vi "QuickDrop Launch Window.vi"(10 "VI":string, 11 "App Refnum":refnum<vi>) -> ()   [LabVIEW 2018]
uses:
  <vilib>/Utility/QuickDropSupport/QuickDrop Plugin Data ver1.ctl
  <vilib>/Utility/miscctls.llb/LVRectTypeDef.ctl
  <vilib>/event_ctls.llb/eventvkey.ctl
  QuickDrop Shortcut Config.vi
  <resource>/dialog/lvconfig.llb/LV Config Write String.vi
  <resource>/dialog/lvconfig.llb/LV Config Read String.vi
  <helpdir>/_LaunchHelp.vi
  Find Project Items.vi
  <resource>/dialog/lvconfig.llb/LV Config Read Boolean.vi
  QuickDrop Get QDKS Mappings.vi
  <vilib>/UDC/API_Files/UDCCountUsage.vi
  <vilib>/UDC/niceiplib.lvlib
  <resource>/dialog/lvconfig.llb/LV Config Write Boolean.vi
  Load Default QD Object Shortcuts.vi
  <vilib>/UDC/API_Files/UDCLogFeatureUsage.vi
panel:
  in  "Object Name":string(combo)
  out "context help name":string
  in  "Waiting Msg":string[](array[string])=["Populating List... Please Wait"]
  out "Shortcuts":string[](array[string])
  in  "Done":bool
  in  "Name Match List":i32(listbox)
  in  "Help":bool
  in  "Configure":bool
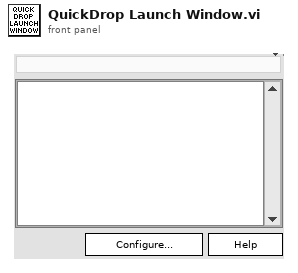
[diagram p1: front panel]
types:
  T1 = enum32{"Invalid", "Standard", "Closed", "Hidden", "Minimized", "Maximized"}
  T2 = cluster{"Left":i16, "Top":i16, "Right":i16, "Bottom":i16}
  T3 = typedef "LVAllMonitorsDisplayTypeDef.ctl" = cluster{"Bounds":cluster{"Left":i16, "Top":i16, "Right":i16, "Bottom":i16}, "Depth":i16}[]
  T4 = typedef "QuickDrop Plugin Data ver1.ctl" = cluster{"FP.IsFrontMost?":bool, "Project VI Path":path, "Palette Object Name":string}
  T5 = typedef "LVRectTypeDef.ctl" = cluster{"Left":i16, "Top":i16, "Right":i16, "Bottom":i16}
  T6 = typedef "eventvkey.ctl" = enum16{"ASCII", "Enter", "Return", "Shift", "Ctrl", "Alt", "Cmd", "Opt", "Caps", "NumLock", "Clear", "Break", "Up", "Down", "Left", "Right", "Insert", "Delete", "Home", "End", "PageUp", "PageDown", "Escape", "Help", "Pause", "ScrollLock", "F1", "F2", "F3", "F4", "F5", "F6", "F7", "F8", "F9", "F10", "F11", "F12", "F13", "F14", "F15", "F16", "F17", "F18", "F19", "F20", "F21", "F22", "F23", "F24", "Play", "VolumeUp", "VolumeDown", "Mute", "Two Byte Char"}
  T7 = cluster{"Shift":bool, "Ctrl":bool, "Alt":bool, "Cmd":bool, "Opt":bool}
  T8 = typedef "LVPoint32TypeDef.ctl" = cluster{"Horizontal":i32, "Vertical":i32}
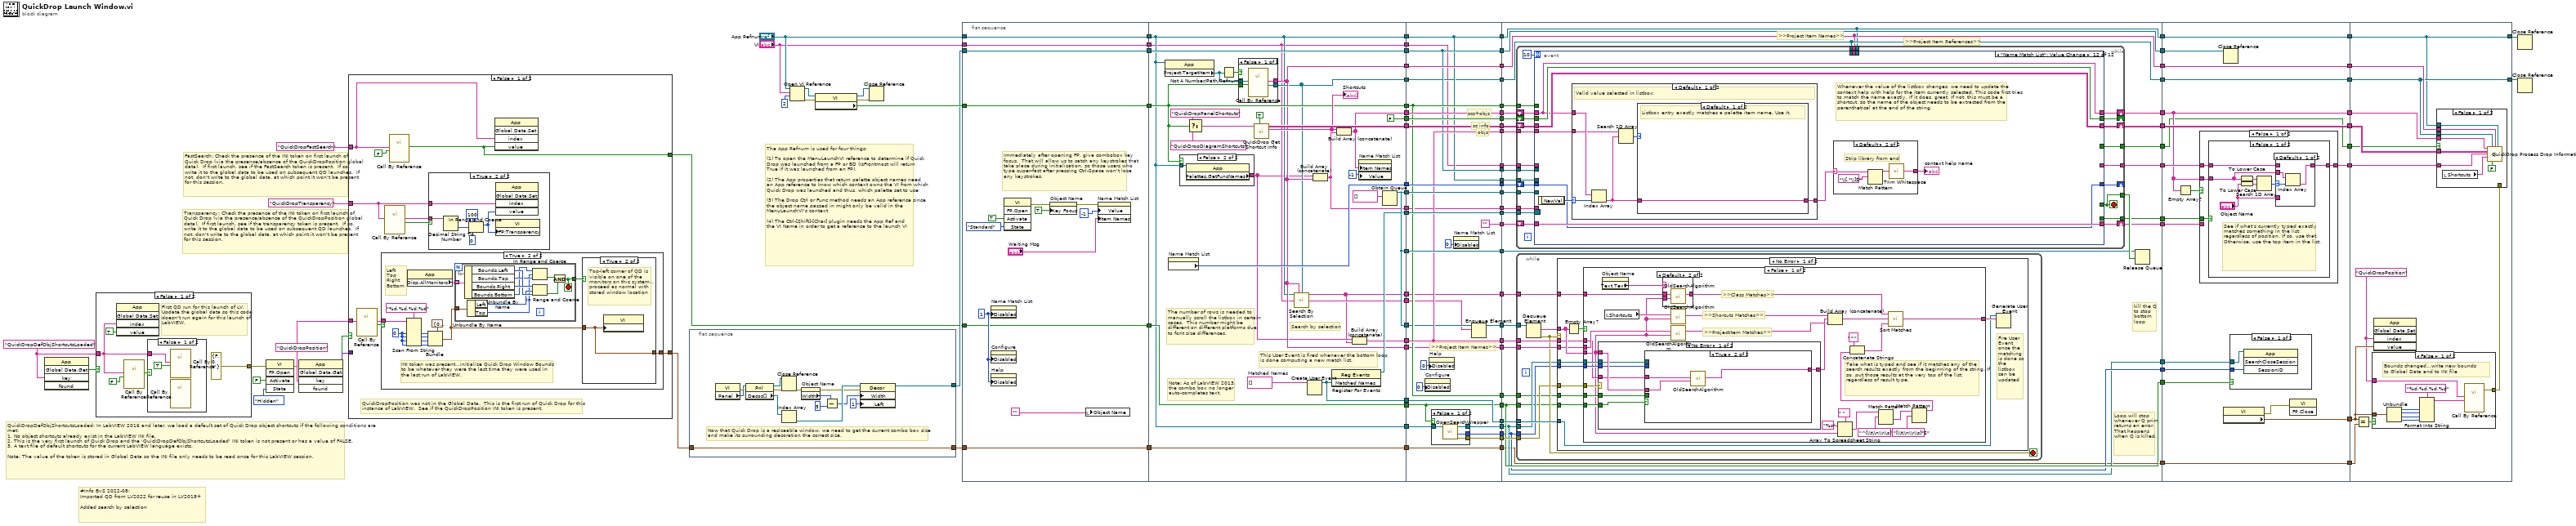
[diagram p0: block diagram]
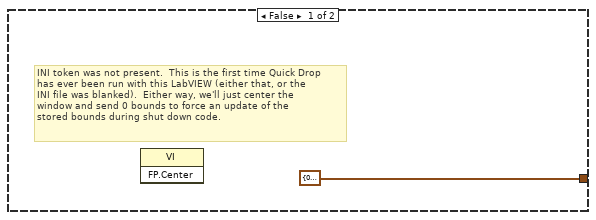
[diagram p5: hidden frame]
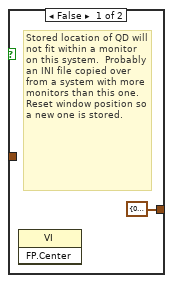
[diagram p6: hidden frame]
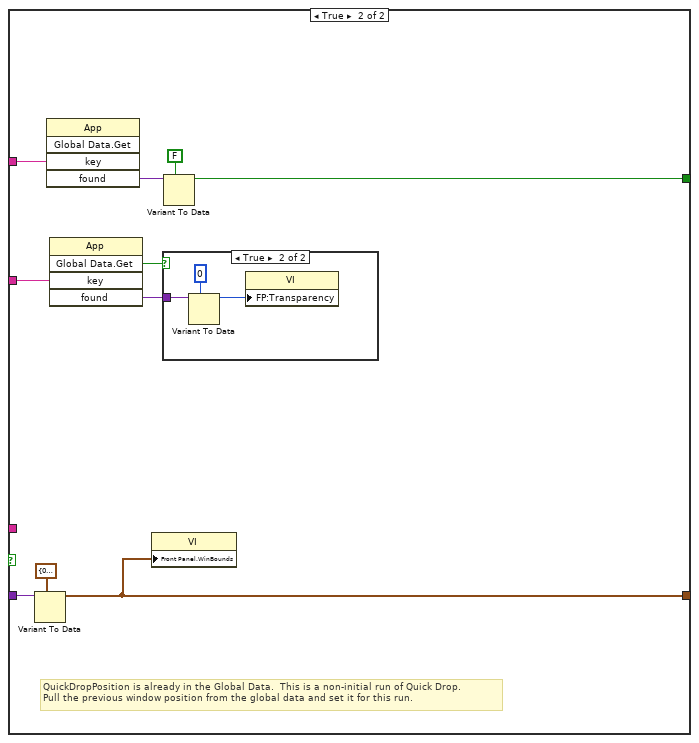
[diagram p7: hidden frame]
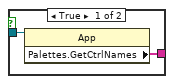
[diagram p10: hidden frame]
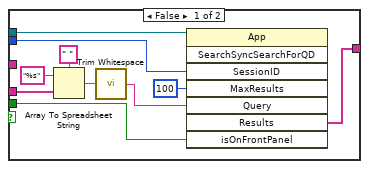
[diagram p13: hidden frame]
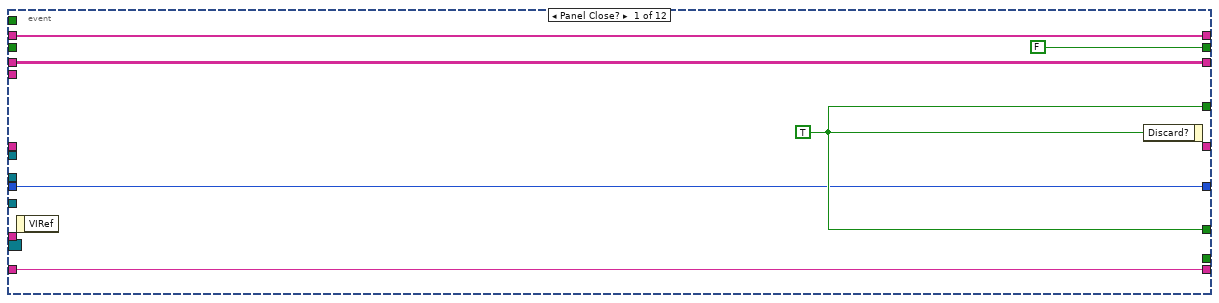
[diagram p17: hidden frame]
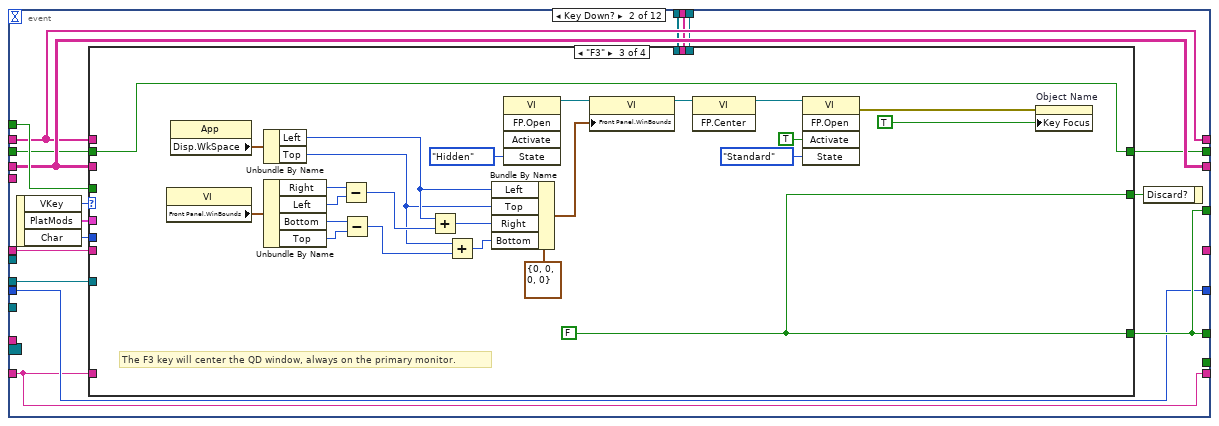
[diagram p18: hidden frame]
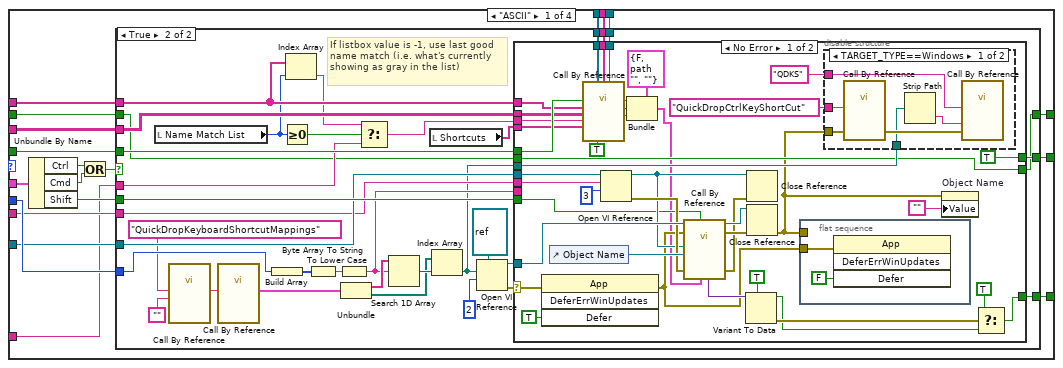
[diagram p19: hidden frame]
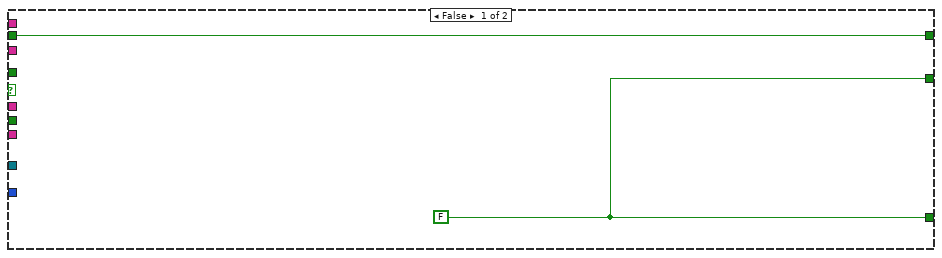
[diagram p20: hidden frame]
diagram:
  w6 = "QuickDropDefObjShortcutsLoaded" ("Name")
  w63 = "QuickDropPosition" ("Name")
  # "#Info BvS 2022-08:\nImported QD from LV2022 for reuse in LV2018+\n\nAdded search by selection"
  # "QuickDropDefObjShortcutsLoaded: In LabVIEW 2016 and later, we load a default set of Quick Drop object shortcuts if the following conditions are met:\n1. No object shortcuts already exist in the LabVIEW INI file.\n2. This is the very first launch of Quick Drop and the 'QuickDropDefObjShortcutsLoaded' INI token is not present or has a value of FALSE.\n3. A text file of default shortcuts for the current LabVIEW language exists.\n\nNote: The value of the token is stored in Global Data so the INI file only needs to be read once for this LabVIEW session."
  # "FastSearch: Check the presence of the INI token on first launch of Quick Drop (via the presence/absence of the QuickDropPosition global data).  If first launch, see if the FastSearch token is present.  If so, write it to the global data to be used on subsequent QD launches.  If not, don't write to the global data, at which point it won't be present for this session."
  # "Transparency: Check the presence of the INI token on first launch of Quick Drop (via the presence/absence of the QuickDropPosition global data).  If first launch, see if the transparency token is present.  If so, write it to the global data to be used on subsequent QD launches.  If not, don't write to the global data, at which point it won't be present for this session."
  # "The App Refnum is used for four things:\n\n(1) To open the MenuLaunchVI reference to determine if Quick Drop was launched from a FP or BD (IsFrontmost will return True if it was launched from an FP).\n\n(2) The App properties that return palette object names need an App reference to know which context owns the VI from which Quick Drop was launched and thus, which palette set to use\n\n(3) The Drop Ctrl or Func method needs an App reference since the object name passed in might only be valid in the MenuLaunchVI's context \n\n(4) The Ctrl-[Shift]-[Char] plugin needs the App Ref and\nthe VI Name in order to get a reference to the launch VI"
  n1 = invoke class="App" method="Global Data.Get"("key"=w6) -> ("GlobalData:Get"=w5:bool)  [unwired: 4 in, 4 out]
  n2 = case shown="False" w5 {
    tunnel: w6 -> [w107 _]
    tunnel: [errorcluster {"status"=FALSE, "code"=0, "source"=""} ("error constant") _] -> w4
    frame False {
      # "First QD run for this launch of LV. Update the global data so this code doesn't run again for this launch of LabVIEW."
      n3 = invoke class="App" method="Global Data.Set"("index"=w107, "value"=TRUE) -> ()  [unwired: 3 in, 5 out]
      n4 = call-by-ref "?"("default value"=FALSE, "key"=w107) -> ("value"=w109:bool)  [unwired: 5 in, 4 out]
      n5 = case shown="False" w109 {
        tunnel: w107 -> [w113 _]
        frame False {
          n6 = call-by-ref "?"("value"=TRUE, "key"=w113) -> ()  [unwired: 7 in, 3 out]
          n7 = call-by-ref "?"() -> ()  [unwired: 14 in, 2 out]
        }
        frame True {
          # "QD default object shortcut code has already been called once in the history of this LabVIEW. Do nothing."
        }
      }
    }
    frame True {
      # "This is the non-initial use of Quick Drop for this launch of LabVIEW. All the Quick Drop default object shortcut initialization stuff has already happened."
    }
  }
  n8 = invoke class="VI" method="FP.Open"(error in=w4, "Activate"=FALSE ("Activate?"), "State"=T1."Hidden") -> (error out=w26:errorcluster)  [unwired: 2 in, 4 out]
  n9 = invoke class="App" method="Global Data.Get"(error in=w26, "key"=w63) -> ("GlobalData:Get"=w10:bool, "found"=w64:variant)  [unwired: 3 in, 3 out]
  n10 = case shown="False" w10 {
    tunnel: w64 -> [_ w165]
    tunnel: [w123 w163] -> w25
    tunnel: w63 -> [w122 _]
    tunnel: "QuickDropTransparency" ("Name") -> [w117 w162]
    tunnel: "QuickDropFastSearch" ("Name") -> [w116 w159]
    tunnel: [w115 w156] -> w17
    frame False {
      # "QuickDropPosition was not in the Global Data.  This is the first run of Quick Drop for this\ninstance of LabVIEW.  See if the QuickDropPosition INI token is present."
      n11 = call-by-ref "?"("key"=w122) -> ("found?"=w121:bool, "value"=w120:string)  [unwired: 6 in, 3 out]
      n12 = case shown="True" w121 {
        tunnel: [T2 {"Left"=0, "Top"=0, "Right"=0, "Bottom"=0} ("Front Panel.PanelBounds") w131] -> w123
        tunnel: w120 -> [_ w142]
        frame False {
          # "INI token was not present.  This is the first time Quick Drop\nhas ever been run with this LabVIEW (either that, or the\nINI file was blanked).  Either way, we'll just center the\nwindow and send 0 bounds to force an update of the\nstored bounds during shut down code."
          n13 = invoke class="VI" method="FP.Center"() -> ()  [unwired: 3 in, 3 out]
        }
        frame True {
          w140 = i16 0 ("default value 1")
          # "Left\nTop\nRight\nBottom"
          # "INI token was present...initialize Quick Drop Window Bounds\nto be whatever they were the last time they were used in\nthe last run of LabVIEW."
          n14 = Scan From String(format string="%d,%d,%d,%d", input string=w142, default 1=w140, default 2=w140, default 3=w140, default 4=w140) -> (output 1=w139:i16, output 2=w138:i16, output 3=w137:i16, output 4=w136:i16)  [unwired: 2 in, 3 out]
          n15 = property class="App"() -> ("Disp.AllMonitors"=w134:T3)  [unwired: 2 in, 2 out]
          n16 = Bundle(cluster=T2 {"Left"=0, "Top"=0, "Right"=0, "Bottom"=0} ("Front Panel.PanelBounds"), "Left"=w139, "Top"=w138, "Right"=w137, "Bottom"=w136) -> (w133:T2)
          n17 = for {
            tunnel: w134 -> [w155] mode=indexing
            tunnel: w133 -> [w154]
            tunnel: [w145] -> w132
            stop <- w145 stop-if-true
            n18 = Unbundle By Name(w155) -> ("Bounds.Left"=w152:i16, "Bounds.Top"=w150:i16, "Bounds.Right"=w153:i16, "Bounds.Bottom"=w149:i16)
            n19 = Unbundle By Name(w154) -> ("Left"=w151:i16, "Top"=w148:i16)
            n20 = In Range and Coerce(upper limit=w149, x=w148, lower limit=w150) -> (In Range?=w147:bool)  [unwired: 1 out]
            n21 = In Range and Coerce(upper limit=w153, x=w151, lower limit=w152) -> (In Range?=w146:bool)  [unwired: 1 out]
            n22 = And(x=w147, y=w146) -> (x .and. y?=w145:bool)
          }
          n23 = case shown="True" w132 {
            tunnel: w133 -> [_ w144]
            tunnel: [T2 {"Left"=0, "Top"=0, "Right"=0, "Bottom"=0} ("Front Panel.PanelBounds") w144] -> w131
            frame False {
              # "Stored location of QD will not fit within a monitor on this system.  Probably an INI file copied over from a system with more monitors than this one.  Reset window position so a new one is stored."
              n24 = invoke class="VI" method="FP.Center"() -> ()  [unwired: 3 in, 3 out]
            }
            frame True {
              # "Top-left corner of QD is visible on one of the monitors on this system... proceed as normal with stored window location"
              n25 = property class="VI"("Front Panel.WinBounds"=w144) -> ()  [unwired: 2 in, 2 out]
            }
          }
        }
      }
      n26 = call-by-ref "?"("key"=w117) -> ("found?"=w119:bool, "value"=w118:string)  [unwired: 6 in, 3 out]
      n27 = call-by-ref "?"("default value"=FALSE, "key"=w116) -> ("value"=w115:bool)  [unwired: 5 in, 4 out]
      n28 = case shown="True" w119 {
        tunnel: w118 -> [_ w129]
        tunnel: w117 -> [_ w125]
        frame False {
        }
        frame True {
          n29 = Decimal String To Number(string=w129) -> (number=w128:i32)  [unwired: 2 in, 1 out]
          n30 = In Range and Coerce(upper limit=100 ("lower limit"), x=w128, lower limit=0) -> (coerced(x)=w124:i32)  [unwired: 1 out]
          n31 = invoke class="App" method="Global Data.Set"("index"=w125, "value"=w124) -> ()  [unwired: 3 in, 5 out]
          n32 = property class="VI"("FP:Transparency"=w124) -> ()  [unwired: 2 in, 2 out]
        }
      }
      n33 = invoke class="App" method="Global Data.Set"("index"=w116, "value"=w115) -> ()  [unwired: 3 in, 5 out]
    }
    frame True {
      # "QuickDropPosition is already in the Global Data.  This is a non-initial run of Quick Drop.\nPull the previous window position from the global data and set it for this run."
      n34 = Variant To Data(type=T2 {"Left"=0, "Top"=0, "Right"=0, "Bottom"=0} ("Front Panel.PanelBounds"), Variant=w165) -> (data=w163:T2)  [unwired: 1 in, 1 out]
      n35 = invoke class="App" method="Global Data.Get"("key"=w159) -> ("found"=w158:variant)  [unwired: 4 in, 4 out]
      n36 = invoke class="App" method="Global Data.Get"("key"=w162) -> ("GlobalData:Get"=w161:bool, "found"=w160:variant)  [unwired: 4 in, 3 out]
      n37 = property class="VI"("Front Panel.WinBounds"=w163) -> ()  [unwired: 2 in, 2 out]
      n38 = case shown="True" w161 {
        tunnel: w160 -> [_ w168]
        frame False {
        }
        frame True {
          n39 = Variant To Data(type=0 ("lower limit"), Variant=w168) -> (data=w166:i32)  [unwired: 1 in, 1 out]
          n40 = property class="VI"("FP:Transparency"=w166) -> ()  [unwired: 2 in, 2 out]
        }
      }
      n41 = Variant To Data(type=FALSE, Variant=w158) -> (data=w156:bool)  [unwired: 1 in, 1 out]
    }
  }
  n42 = flat-sequence {
    tunnel: [w182] -> w24
    tunnel: w25 -> [w182]
    tunnel: [w170] -> w23
    frame #0 {
      # "Now that Quick Drop is a resizeable window, we need to get the current combo box size\nand make its surrounding decoration the correct size."
      n43 = property class="VI"() -> (error out=w171:errorcluster, "Panel"=w172:refnum<vi>)  [unwired: 2 in, 1 out]
      n44 = property class="Pnl"(reference=w172, error in=w171) -> (reference out=w174:refnum<vi>, error out=w173:errorcluster, "Decos[]"=w179:refnum<vi>[])
      n45 = Index Array(array=w179) -> (element=w181:refnum<vi>)  [unwired: 1 in]
      n46 = Close Reference(reference=w174, error in (no error)=w173) -> (error out=w175:errorcluster)
      n47 = property on="Object Name" class="CmbBox"(error in=w175) -> (error out=w180:errorcluster, "Width"=w176:u32)  [unwired: 1 in, 1 out]
      n48 = Subtract(x=w176, y=u32 5) -> (x-y=w178:u32)
      n49 = property class="Decor"(reference=w181, error in=w180, "Width"=w178, "Left"=1 ("Position:Left")) -> (reference out=w170:refnum<vi>)  [unwired: 1 out]
    }
  }
  n50 = Open VI Reference(application reference (local)="App Refnum", vi path="VI", options=2) -> (vi reference=w75:refnum<vi>, error out=w65:errorcluster)  [unwired: 1 in, 2 out]
  n51 = property class="VI"(reference=w75, error in=w65) -> (reference out=w73:refnum<vi>, error out=w74:errorcluster, "Front Panel.IsFrontmost"=w72:bool)
  n52 = Close Reference(reference=w73, error in (no error)=w74) -> ()  [unwired: 1 out]
  n53 = flat-sequence {
    tunnel: w24 -> [w195]
    tunnel: w72 -> [w196]
    tunnel: "App Refnum" -> [w197]
    tunnel: [w197] -> w54
    tunnel: [w196] -> w53
    tunnel: [w195] -> w52
    tunnel: [w189] -> w35
    tunnel: "VI" -> [w189]
    tunnel: [w185] -> w29
    tunnel: w23 -> [w185]
    tunnel: [w184] -> w18
    tunnel: w17 -> [w184]
    tunnel: [w216] -> w106
    tunnel: [FALSE] -> w104
    tunnel: [w226] -> w102
    tunnel: [w226] -> w100
    tunnel: [w205] -> w98
    tunnel: [w226] -> w96
    tunnel: [w201] -> w94
    tunnel: [w224] -> w92
    tunnel: [w223] -> w90
    tunnel: [w222] -> w88
    tunnel: [w210] -> w84
    tunnel: [w217] -> w82
    tunnel: [w203] -> w70
    tunnel: [w213] -> w62
    tunnel: w54 -> [w203]
    tunnel: w53 -> [w210]
    tunnel: w52 -> [w213]
    tunnel: [w204] -> w50
    tunnel: [w205] -> w46
    tunnel: [w203] -> w42
    tunnel: w35 -> [w202]
    tunnel: [w202] -> w32
    tunnel: [w209] -> w30
    tunnel: w29 -> [w208]
    tunnel: [w208] -> w28
    tunnel: w18 -> [w207]
    tunnel: [w207] -> w15
    tunnel: [w198] -> w2
    tunnel: [w199] -> w1
    tunnel: w106 -> [w266]
    tunnel: [w266] -> w105
    tunnel: w104 -> [w265]
    tunnel: [w265] -> w103
    tunnel: w102 -> [w264]
    tunnel: [w264] -> w101
    tunnel: w100 -> [w243]
    tunnel: [w242] -> w99
    tunnel: w98 -> [w240]
    tunnel: [w240] -> w97
    tunnel: w96 -> [w263]
    tunnel: [w263] -> w95
    tunnel: w94 -> [w259]
    tunnel: [w259] -> w93
    tunnel: w92 -> [w262]
    tunnel: [w262] -> w91
    tunnel: w90 -> [w246]
    tunnel: [w246] -> w89
    tunnel: w88 -> [w261]
    tunnel: [w261] -> w87
    tunnel: [w259] -> w86
    tunnel: [w249] -> w85
    tunnel: w84 -> [w249]
    tunnel: [w260] -> w83
    tunnel: w82 -> [w260]
    tunnel: [w241] -> w71
    tunnel: w70 -> [w241]
    tunnel: [w241] -> w67
    tunnel: w62 -> [w258]
    tunnel: [w258] -> w59
    tunnel: w50 -> [w239]
    tunnel: [w239] -> w49
    tunnel: w46 -> [w254]
    tunnel: [w254] -> w45
    tunnel: w42 -> [w253]
    tunnel: [w252] -> w41
    tunnel: [w251] -> w40
    tunnel: [w250] -> w39
    tunnel: [w249] -> w38
    tunnel: [w238] -> w33
    tunnel: w32 -> [w238]
    tunnel: [w248] -> w31
    tunnel: w30 -> [w248]
    tunnel: w28 -> [w247]
    tunnel: [w247] -> w27
    tunnel: [w247] -> w21
    tunnel: [w245] -> w16
    tunnel: w15 -> [w245]
    tunnel: [""] -> w9
    tunnel: [w237] -> w3
    tunnel: w2 -> [w237]
    tunnel: w1 -> [w236]
    tunnel: w105 -> [w306]
    tunnel: w103 -> [w305]
    tunnel: w101 -> [w304]
    tunnel: w99 -> [w303]
    tunnel: w97 -> [w302]
    tunnel: w95 -> [w300]
    tunnel: w93 -> [w299]
    tunnel: w91 -> [w298]
    tunnel: w89 -> [w297]
    tunnel: w87 -> [w296]
    tunnel: [w295] -> w81
    tunnel: [w294] -> w79
    tunnel: w86 -> [w293]
    tunnel: w85 -> [w292]
    tunnel: w83 -> [w291]
    tunnel: [w290] -> w77
    tunnel: w71 -> [w275]
    tunnel: [w275] -> w68
    tunnel: w67 -> [w289]
    tunnel: [w279] -> w60
    tunnel: w59 -> [w279]
    tunnel: [w288] -> w55
    tunnel: w49 -> [w277]
    tunnel: [w277] -> w48
    tunnel: w45 -> [w276]
    tunnel: [w276] -> w44
    tunnel: w41 -> [w280]
    tunnel: w40 -> [w281]
    tunnel: w39 -> [w287]
    tunnel: w38 -> [w286]
    tunnel: [w280] -> w37
    tunnel: [w281] -> w36
    tunnel: w33 -> [w285]
    tunnel: w31 -> [w284]
    tunnel: w27 -> [w283]
    tunnel: [w278] -> w22
    tunnel: w21 -> [w278]
    tunnel: w16 -> [w282]
    tunnel: [w282] -> w14
    tunnel: w9 -> [w274]
    tunnel: [w273] -> w8
    tunnel: [w272] -> w7
    tunnel: w3 -> [w271]
    tunnel: w81 -> [w908]
    tunnel: [w908] -> w80
    tunnel: w79 -> [w911]
    tunnel: [w910] -> w78
    tunnel: w77 -> [w922]
    tunnel: [w922] -> w76
    tunnel: [w921] -> w69
    tunnel: w68 -> [w921]
    tunnel: [w920] -> w61
    tunnel: w60 -> [w920]
    tunnel: [w919] -> w58
    tunnel: w55 -> [w909]
    tunnel: w48 -> [w917]
    tunnel: [w917] -> w47
    tunnel: w44 -> [w916]
    tunnel: [w916] -> w43
    tunnel: w37 -> [w915]
    tunnel: w36 -> [w914]
    tunnel: w22 -> [w913]
    tunnel: w14 -> [w912]
    tunnel: [w909] -> w13
    tunnel: w8 -> [w906]
    tunnel: w7 -> [w905]
    tunnel: w80 -> [w948]
    tunnel: w78 -> [w953]
    tunnel: w76 -> [w952]
    tunnel: w69 -> [w944]
    tunnel: w61 -> [w951]
    tunnel: w58 -> [w943]
    tunnel: w47 -> [w945]
    tunnel: w43 -> [w949]
    tunnel: w13 -> [w946]
    tunnel: [w945] -> w12
    tunnel: [w944] -> w11
    frame #0 {
      w191 = u8 1 ("Disabled")
      # "Immediately after opening FP, give combobox key focus.  That will allow us to catch any keystrokes that take place during initialization, so those users who type super-fast after pressing Ctrl-Space won't lose any keystrokes."
      n54 = property on="Name Match List" class="LstBox (strict)"("Disabled"=w191) -> ()  [unwired: 2 in, 2 out]
      n55 = property on="Configure" class="Bool"("Disabled"=w191) -> ()  [unwired: 2 in, 2 out]
      n56 = property on="Help" class="Bool"("Disabled"=w191) -> ()  [unwired: 2 in, 2 out]
      n57 = invoke class="VI" method="FP.Open"("Activate"=TRUE ("Activate?"), "State"=T1."Standard") -> (error out=w187:errorcluster)  [unwired: 3 in, 4 out]
      n58 = property on="Object Name" class="CmbBox"(error in=w187, "Key Focus"=TRUE) -> (error out=w186:errorcluster)  [unwired: 1 in, 1 out]
      n59 = local write "Object Name"("") -> ()
      n60 = property on="Name Match List" class="LstBox (strict)"(error in=w186, "Value"=-1 ("Name Match List"), "Item Names"="Waiting Msg") -> ()  [unwired: 1 in, 2 out]
    }
    frame #1 {
      w225 = string[] []  # Matched Names
      # "Search by selection"
      # "Note: As of LabVIEW 2013,\nthe combo box no longer\nauto-completes text."
      # "The number of rows is needed to manually scroll the listbox in certain cases.  This number might be different on different platforms due to font size differences."
      # "This User Event is fired whenever the bottom loop is done computing a new match list."
      n61 = property class="App"(reference=w203) -> ("Project.TargetItem"=w206:refnum<vi>)  [unwired: 1 in, 2 out]
      n62 = property on="Name Match List" class="LstBox (strict)"() -> ("Number of Rows"=w222:u32)  [unwired: 2 in, 2 out]
      n63 = case shown="False" w210 {
        tunnel: [w233 w235] -> w200
        tunnel: w203 -> [w232 w234]
        frame True {
          n64 = property class="App"(reference=w232) -> ("Palettes.GetCtrlNames"=w233:string[])  [unwired: 1 in, 2 out]
        }
        frame False {
          n65 = property class="App"(reference=w234) -> ("Palettes.GetFuncNames"=w235:string[])  [unwired: 1 in, 2 out]
        }
      }
      n66 = Select(t="QuickDropPanelShortcuts" ("Name"), s=w210, f="QuickDropDiagramShortcuts" ("Name")) -> (s? t:f=w219:string)
      n67 = Not A Number/Path/Refnum?(number/path/refnum=w206) -> (NaN/Path/Refnum?=w211:bool)
      n68 = case shown="False" w211 {
        tunnel: w206 -> [w228 _]
        tunnel: w210 -> [w231 _]
        tunnel: [w230 _] -> w205
        tunnel: [w229 _] -> w204
        frame False {
          n69 = call-by-ref "?"("Panel?"=w231, "Target Item"=w228) -> ("Project Item Ref"=w229:refnum<vi>[], "Hierarchy"=w230:string[])  [unwired: 10 in, 2 out]
        }
        frame True {
        }
      }
      n70 = call "QuickDrop Get Shortcut Info.vi"("Generate Listbox Strings?"=TRUE, "Shortcut Type"=w219) -> ("Listbox Strings"=w215:string[], "Shortcut Info"=w217:string[][])  [unwired: 1 in, 7 out]
      "Shortcuts" <- w215
      n71 = call "Search By Selection.vi"("App Refnum"=w203, "Project Item Names"=w205, "Project Item Refs"=w204, "VI"=w202) -> ("Class Item Names"=w198:string[], "Query terms"=w199:string[])  [unwired: 9 in, 1 out]
      n72 = Create User Event(user event datatype=w225) -> (user event=w223:refnum<user-event>)  [unwired: 1 in, 1 out]
      n73 = Build Array (concatenate)(w200, w205) -> (w209:string[])
      n74 = register-events(w223) -> (reference out=w224:refnum<event-registration>)  [unwired: 2 in, 1 out]
      n75 = Build Array (concatenate)(w215, w209) -> (w216:string[])
      n76 = Build Array (concatenate)(w200, w198) -> (w201:string[])
      n77 = property on="Name Match List" class="LstBox (strict)"("Item Names"=w216, "Value"=-1 ("Listbox")) -> ()  [unwired: 2 in, 2 out]
      n78 = Obtain Queue(element data type=string[] []) -> (queue out=w226:refnum<queue>)  [unwired: 3 in, 3 out]
    }
    frame #2 {
      # ">>Project Item Names>>"
      # "objs"
      # "sc info"
      # "scs+objs"
      n79 = property on="Configure" class="Bool"("Disabled"=u8 0) -> ()  [unwired: 2 in, 2 out]
      n80 = property on="Help" class="Bool"("Disabled"=u8 0) -> ()  [unwired: 2 in, 2 out]
      n81 = case shown="False" w245 {
        tunnel: w253 -> [w270 _]
        tunnel: [w269 _] -> w252
        tunnel: [w268 _] -> w251
        tunnel: [w267 _] -> w250
        frame False {
          n82 = call "OpenSearchWrapper.vi"("App Refnum"=w270) -> ("error out"=w267:errorcluster, "Session ID out"=w268:u32, "App Refnum Out"=w269:refnum<vi>)  [unwired: 8 in]
        }
        frame True {
        }
      }
      n83 = property on="Name Match List" class="LstBox (strict)"("Disabled"=u8 0) -> ()  [unwired: 2 in, 2 out]
      n84 = Enqueue Element(queue=w243, element=w236) -> (queue out=w242:refnum<queue>)  [unwired: 2 in, 2 out]
    }
    frame #3 {
      # ">>Project Item Names>>"
      # ">>Project Item References>>"
      # "Loop will stop whenever Q prim returns an error.  That happens when Q is killed."
      # "kill the Q\nto stop\nbottom\nloop"
      n85 = while {
        shift-right: [w406] -> w288
        shift-left: w306 -> [w407]
        shift-right: [w403] -> _
        shift-left: w305 -> [w404]
        tunnel: w304 -> [w402]
        tunnel: [w401] -> w301
        tunnel: w298 -> [w400]
        tunnel: [w398] -> w295
        tunnel: [w397] -> w294
        tunnel: w293 -> [w396]
        tunnel: w292 -> [w395]
        shift-right: [w393] -> w290
        shift-left: w291 -> [w394]
        tunnel: w289 -> [w392]
        tunnel: w285 -> [w391]
        tunnel: w284 -> [w390]
        tunnel: w283 -> [w389]
        shift-right: [w388] -> _
        shift-left: w296 -> [w399]
        tunnel: w277 -> [w387]
        tunnel: w276 -> [w386]
        tunnel: w275 -> [w385]
        shift-right: [w383] -> w273
        shift-left: w274 -> [w384]
        tunnel: [w382] -> w272
        stop <- w401 stop-if-true
        n86 = event shown="[11] \"Name Match List\": Value Change" {
          selector: w400 -> [_ _ _ _ _ _ _ _ _ _ _ _]
          dyn-events: _ -> [_ _ _ _ _ _ _ _ _ _ _ _]
          timeout: 10 -> [_ _ _ _ _ _ _ _ _ _ _ _]
          tunnel: [w411 w430 TRUE ("Discard?") w591 w609 _ _ _ _ _ _ _] -> w401
          tunnel: w407 -> [w413 w420 w579 w590 w602 w620 w626 w660 w793 _ w876 w880]
          tunnel: [w413 w420 w579 w590 w602 w620 w625 w660 w793 w820 w876 w880] -> w406
          tunnel: w404 -> [_ w415 _ _ _ w619 _ _ w790 w815 w875 w883]
          tunnel: [FALSE w414 FALSE FALSE FALSE w619 FALSE w648 FALSE w815 w875 w883] -> w403
          tunnel: w402 -> [_ _ _ _ _ _ _ _ w791 _ _ _]
          tunnel: w399 -> [w409 w424 w580 w586 w605 w615 w623 w659 w788 w828 _ w879]
          tunnel: [w411 w430 FALSE ("Discard?") FALSE ("Discard?") FALSE ("Discard?") _ _ _ _ _ _ _] -> w398
          tunnel: [_ _ w578 w595 w603 _ _ _ _ _ _ _] -> w397
          tunnel: w396 -> [_ _ _ _ _ _ w632 _ _ _ _ w881]
          tunnel: w395 -> [_ w423 _ _ _ _ w633 _ _ _ _ _]
          tunnel: w394 -> [w410 w421 w581 w596 w606 w618 w627 w662 w789 w821 w874 w882]
          tunnel: [w410 w421 w581 w596 w606 w618 w629 w662 w789 w821 w874 w882] -> w393
          tunnel: w392 -> [_ w426 _ _ _ _ w630 _ _ _ _ _]
          tunnel: w391 -> [_ w425 _ _ _ _ _ _ _ _ _ _]
          tunnel: w390 -> [_ _ _ _ _ _ w624 _ _ _ _ _]
          tunnel: w389 -> [_ _ _ _ _ _ _ _ _ _ w870 _]
          tunnel: [w409 w424 w580 w586 w605 w615 w623 w659 w788 w828 w867 w879] -> w388
          tunnel: w387 -> [_ w419 _ _ _ _ _ _ _ _ _ _]
          tunnel: w386 -> [_ w418 _ _ _ _ _ _ _ _ _ _]
          tunnel: w385 -> [_ w417 _ _ _ _ _ _ _ _ _ _]
          tunnel: w384 -> [w408 w416 w577 w585 w601 w614 w622 w649 w787 w826 w865 w885]
          tunnel: [w408 w416 w577 w585 w601 w614 w622 w649 w787 w816 w865 w885] -> w383
          tunnel: [_ _ w575 w584 w599 _ _ _ _ _ _ _] -> w382
          event Panel Close? {
            w411 = TRUE ("Discard?")
            n87 = event-data() -> ()  [unwired: 2 out]
            n88 = event-data("Discard?"=w411) -> ()  [unwired: 1 in, 1 out]
          }
          event Key Down? {
            n89 = event-data() -> ("VKey"=w429:T6, "PlatMods"=w428:T7, "Char"=w427:i16)  [unwired: 1 out]
            n90 = case shown="\"F3\"" w429 {
              tunnel: [w444 TRUE w571 w573] -> w430
              tunnel: w428 -> [w449 _ _ _]
              tunnel: w427 -> [w443 _ _ _]
              tunnel: w426 -> [w442 _ _ _]
              tunnel: w425 -> [w441 _ _ _]
              tunnel: w423 -> [w440 _ _ _]
              tunnel: [w439 FALSE w571 w573] -> w422
              tunnel: w421 -> [w438 _ _ _]
              tunnel: w420 -> [w437 _ _ _]
              tunnel: w419 -> [w436 _ _ _]
              tunnel: w418 -> [w435 _ _ _]
              tunnel: w417 -> [w434 _ _ _]
              tunnel: w416 -> [w433 _ _ _]
              tunnel: w415 -> [w432 w545 w548 w572]
              tunnel: [w431 w545 w548 w572] -> w414
              frame "ASCII" {
                n91 = Unbundle By Name(w449) -> ("Ctrl"=w448:bool, "Cmd"=w447:bool, "Shift"=w445:bool)
                n92 = Or(x=w448, y=w447) -> (x .or. y?=w446:bool)
                n93 = case shown="True" w446 {
                  tunnel: w445 -> [_ w480]
                  tunnel: [w451 w481] -> w444
                  tunnel: w443 -> [_ w465]
                  tunnel: w442 -> [_ w479]
                  tunnel: w441 -> [_ w478]
                  tunnel: w440 -> [_ w477]
                  tunnel: [w451 w476] -> w439
                  tunnel: w438 -> [_ w471]
                  tunnel: w437 -> [_ w466]
                  tunnel: w436 -> [_ w469]
                  tunnel: w435 -> [_ w468]
                  tunnel: w434 -> [_ w467]
                  tunnel: w433 -> [_ w456]
                  tunnel: w432 -> [w450 w453]
                  tunnel: [w450 w452] -> w431
                  frame False {
                    w451 = FALSE
                  }
                  frame True {
                    # "If listbox value is -1, use last good name match (i.e. what's currently showing as gray in the list)"
                    n94 = local read "Name Match List"() -> (w459:i32)
                    n95 = call-by-ref "?"("default value"="", "key"="QuickDropKeyboardShortcutMappings" ("Name")) -> ("value"=w464:string)  [unwired: 5 in, 4 out]
                    n96 = call-by-ref "?"("Mappings from INI"=w464) -> ("Key to VI Mappings"=w462:cluster{"Keys":string[], "VIs":path[]})  [unwired: 11 in, 3 out]
                    n97 = Build Array(w465) -> (w486:i16[])
                    n98 = Greater Or Equal To 0?(x=w459) -> (x >= 0?=w460:bool)
                    n99 = Index Array(array=w466, index=w459) -> (element=w458:string)
                    n100 = Byte Array To String(unsigned byte array=w486) -> (string=w475:string)
                    n101 = To Lower Case(string=w475) -> (all lower case string=w455:string)
                    n102 = Unbundle(w462) -> ("Keys"=w474:string[], "VIs"=w472:path[])
                    n103 = Select(t=w458, s=w460, f=w456) -> (s? t:f=w457:string)
                    n104 = Search 1D Array(1D array=w474, element=w455) -> (index of element=w473:i32)  [unwired: 1 in]
                    n105 = local read "Shortcuts"() -> (w470:string[])
                    n106 = Index Array(array=w472, index=w473) -> (element=w454:path)
                    n107 = Open VI Reference(type specifier VI Refnum (for type only)=refnum<vi> refnum, vi path=w454, options=2) -> (vi reference=w483:refnum<vi>, error out=w484:errorcluster)  [unwired: 3 in]
                    n108 = case shown="No Error" w484 {
                      selector: w484 -> [w491 _]
                      tunnel: w483 -> [w526 _]
                      tunnel: [w511 FALSE] -> w481
                      tunnel: w480 -> [w517 _]
                      tunnel: w479 -> [w522 _]
                      tunnel: w478 -> [w521 _]
                      tunnel: w477 -> [w507 _]
                      tunnel: [TRUE w537] -> w476
                      tunnel: w471 -> [w504 _]
                      tunnel: w470 -> [w503 _]
                      tunnel: w457 -> [w502 _]
                      tunnel: w466 -> [w501 _]
                      tunnel: w469 -> [w500 _]
                      tunnel: w468 -> [w499 _]
                      tunnel: w467 -> [w498 _]
                      tunnel: w455 -> [_ w538]
                      tunnel: w454 -> [w494 _]
                      tunnel: w453 -> [w492 w536]
                      tunnel: [w492 w535] -> w452
                      frame No Error {
                        n109 = invoke class="App" method="DeferErrWinUpdates"(error in=w491, "Defer"=TRUE) -> (error out=w488:errorcluster)  [unwired: 2 in, 3 out]
                        n110 = control-ref of="Object Name"() -> (w523:refnum<vi>)
                        n111 = call-by-ref "?"("Listbox Contents"=w501, "Project Item Refs"=w500, "Project Items"=w499, "App Refnum"=w498, "Shortcut Info"=w504, "Text.Text"=w502, "Shortcuts"=w503, "Run for Plugin?"=TRUE) -> ("Project VI Path"=w506:path, "Palette Object Name"=w497:string)  [unwired: 8 in, 2 out]
                        n112 = Open VI Reference(application reference (local)=w522, vi path=w521, options=3) -> (vi reference=w519:refnum<vi>, error out=w520:errorcluster)  [unwired: 3 in]
                        n113 = Bundle(cluster=T4 {"FP.IsFrontMost?"=FALSE, "Project VI Path"=path "", "Palette Object Name"=""} ("Quick Drop Plugin Data"), "FP.IsFrontMost?"=w507, "Project VI Path"=w506, "Palette Object Name"=w497) -> (w487:T4)
                        n114 = call-by-ref "?"(reference=w526, error in=w488, "Variant in"=w487, "Shift Pressed?"=w517, 8:"error in (no error)"=w520, "QD Combo Box Ref"=w523, "QD Launch VI Ref"=w519) -> (reference out=w524:refnum<vi>, error out=w525:errorcluster, 0:"error out"=w518:errorcluster, "Variant out"=w516:variant)  [unwired: 5 in]
                        n115 = Variant To Data(type=TRUE, Variant=w516) -> (data=w513:bool, error out=w514:errorcluster)  [unwired: 1 in]
                        n116 = Close Reference(reference=w519, error in (no error)=w518) -> ()  [unwired: 1 out]
                        n117 = Close Reference(reference=w524, error in (no error)=w525) -> (error out=w489:errorcluster)
                        n118 = flat-sequence {
                          tunnel: w489 -> [_]
                          tunnel: w488 -> [w528]
                          frame #0 {
                            n119 = invoke class="App" method="DeferErrWinUpdates"(error in=w528, "Defer"=FALSE) -> ()  [unwired: 2 in, 4 out]
                          }
                        }
                        n120 = disable-structure shown="TARGET_TYPE==Windows" {
                          disable-tunnel: "QuickDropCtrlKeyShortCut" -> [w532 _]
                          disable-tunnel: w489 -> [w534 _]
                          disable-tunnel: w494 -> [w531 _]
                          disable-tunnel: "QDKS" -> [w529 _]
                          frame condition #0 (active) {
                            n121 = call-by-ref "?"("Error In"=w534, "CounterName"=w532) -> ("Error Out"=w533:errorcluster)  [unwired: 11 in, 2 out]
                            n122 = Strip Path(path=w531) -> (name=w530:string)  [unwired: 1 out]
                            n123 = call-by-ref "?"("Error In"=w533, "subFeatureName"=w530, "featureName"=w529) -> ()  [unwired: 10 in, 3 out]
                          }
                          frame condition #1 {
                          }
                        }
                        n124 = property on="Object Name" class="CmbBox"(error in=w489, "Value"="") -> ()  [unwired: 1 in, 2 out]
                        n125 = Select(t=TRUE, s=w514, f=w513) -> (s? t:f=w511:bool)
                      }
                      frame Error {
                        # "This might be a Ctrl-A/C/V/X that the user is performing in the text box, so don't discard it if it's not a match for a plugin VI"
                        n126 = case shown="Default" w538 {
                          tunnel: [_ TRUE] -> w537
                          tunnel: w536 -> [_ w541]
                          tunnel: [TRUE w541] -> w535
                          frame Default {
                            # "This may have been Ctrl-X or Ctrl-V, which will affect the contents of the search results, so we should trigger the Timeout case to refresh the search results."
                          }
                          frame "a" {
                            # "The combo box doesn't support Ctrl-A for Select All, so this code implements it instead, as long as there isn't a QDKS for the 'A' key."
                            n127 = property on="Object Name" class="CmbBox"("Text.Selection Start"=u32 0 ("Text.Selection:Start"), "Text.Selection End"=u32 999 ("Text.Selection:End")) -> ()  [unwired: 2 in, 2 out]
                          }
                        }
                      }
                    }
                  }
                }
              }
              frame "Escape" {
                # "Cancel the dialog if Esc is pressed during its use"
              }
              frame "F3" {
                w571 = FALSE
                # "The F3 key will center the QD window, always on the primary monitor."
                n128 = property class="VI"() -> ("Front Panel.WinBounds"=w570:T5)  [unwired: 2 in, 2 out]
                n129 = property class="App"() -> ("Disp.WkSpace"=w565:T5)  [unwired: 2 in, 2 out]
                n130 = Unbundle By Name(w565) -> ("Left"=w554:i16, "Top"=w551:i16)
                n131 = Unbundle By Name(w570) -> ("Right"=w568:i16, "Left"=w569:i16, "Bottom"=w567:i16, "Top"=w566:i16)
                n132 = Subtract(x=w568, y=w569) -> (x-y=w552:i16)
                n133 = Subtract(x=w567, y=w566) -> (x-y=w549:i16)
                n134 = Add(x=w554, y=w552) -> (x+y=w553:i16)
                n135 = Add(x=w551, y=w549) -> (x+y=w550:i16)
                n136 = Bundle By Name(cluster=T5 {"Left"=0, "Top"=0, "Right"=0, "Bottom"=0} ("Front Panel Window:Window Bounds"), "Left"=w554, "Top"=w551, "Right"=w553, "Bottom"=w550) -> (w555:T5)
                n137 = invoke class="VI" method="FP.Open"("State"=T1."Hidden") -> (reference out=w563:refnum<vi>)  [unwired: 4 in, 4 out]
                n138 = property class="VI"(reference=w563, "Front Panel.WinBounds"=w555) -> (reference out=w562:refnum<vi>)  [unwired: 1 in, 1 out]
                n139 = invoke class="VI" method="FP.Center"(reference=w562) -> (reference out=w560:refnum<vi>)  [unwired: 2 in, 2 out]
                n140 = invoke class="VI" method="FP.Open"(reference=w560, "Activate"=TRUE ("Activate?"), "State"=T1."Standard") -> (error out=w557:errorcluster)  [unwired: 2 in, 4 out]
                n141 = property on="Object Name" class="CmbBox"(error in=w557, "Key Focus"=TRUE) -> ()  [unwired: 1 in, 2 out]
              }
              frame Default {
                w573 = FALSE
              }
            }
            n142 = event-data("Discard?"=w422) -> ()  [unwired: 1 in, 1 out]
          }
          event "Done": Value Change {
            # "The Done button is off-screen, but has Enter set for Key Focus.  So if Enter is pressed, it acts like a commit. Pull the first value from the listbox and use that as the object to drop."
            n143 = event-data() -> ()  [unwired: 2 out]
            n144 = Index Array(array=w579, index="Name Match List") -> (element=w578:string)
            n145 = Greater Than 0?(x="Name Match List") -> (x > 0?=w575:bool)
          }
          event "Name Match List": Mouse Up {
            # "Pull the first value from the listbox and use that as the object to drop."
            # "Conditions:\n1.  Mouse Up was not in empty space after the last row.\n2.  Mouse Up was not on scrollbars.\n3.  A valid row is selected in the listbox.\n4.  This was the second Mouse Up from a double click."
            n146 = event-data() -> ("Coords"=w594:T8, "Mods.Double Click"=w584:bool)  [unwired: 1 out]
            n147 = invoke on="Name Match List" class="LstBox (strict)" method="Point To Row"("Point"=w594) -> ("InBounds"=w593:bool, "Row"=w587:i32)  [unwired: 6 in, 5 out]
            n148 = Array Size(array=w590) -> (size(s)=w589:i32)
            n149 = Greater Or Equal To 0?(x=w587) -> (x >= 0?=w592:bool)
            n150 = Greater?(x=w589, y=w587) -> (0:w588:bool)
            n151 = Compound Arithmetic op=AND(w588, w593, w592, w584) -> (w591:bool)
            n152 = Index Array(array=w590, index=w587) -> (element=w595:string)
          }
          event VI Activation {
            # "Pull the first value from the listbox and use that as the object to drop."
            # "Use VI Name property instead of a string constant for advanced customer hacking use case"
            # "If there is a VI Activation event, then the user has clicked outside\nof the Quick Drop window, so act like a commit.  Notice the two exceptions\nare if the Quick Drop window itself or its Shortcut Config dialog are\nactivated...in those cases, don't dismiss Quick Drop."
            n153 = event-data() -> ("VIName"=w610:string)  [unwired: 1 out]
            n154 = property class="VI"() -> ("Name"=w604:string)  [unwired: 2 in, 2 out]
            n155 = Not Equal?(x=w604, y=w610) -> (x != y?=w613:bool)
            n156 = Not Equal?(x=w610, y="QuickDrop Shortcut Config.vi") -> (x != y?=w612:bool)
            n157 = And(x=w613, y=w612) -> (x .and. y?=w609:bool)
            n158 = local read "Name Match List"() -> (w600:i32)
            n159 = Index Array(array=w602, index=w600) -> (element=w603:string)
            n160 = Greater Than 0?(x=w600) -> (x > 0?=w599:bool)
          }
          event "Help": Value Change {
            n161 = event-data() -> ()  [unwired: 2 out]
            n162 = call-by-ref "?"("CHM or HLP filename (lvdialog.chm)"="lvdialog.chm", "HTML filename"="quick_drop_db.html") -> ()  [unwired: 3 in, 7 out]
          }
          event "Configure": Value Change {
            # "Call the Configure dialog dynamically so it doesn't have to load with Quick Drop"
            n163 = event-data() -> ()  [unwired: 2 out]
            n164 = call-by-ref "?"("App.MenuLaunchApp"=w630, "Shortcut Info in"=w627, "Retrieved Obj Names"=w632, "Panel?"=w633) -> ("Shortcut Info out"=w631:string[][], "Changes?"=w628:bool)  [unwired: 2 in, 8 out]
            n165 = case shown="True" w628 {
              tunnel: w624 -> [_ w642]
              tunnel: w631 -> [_ w641]
              tunnel: [w635 w641] -> w629
              tunnel: w627 -> [w635 _]
              tunnel: w626 -> [w634 _]
              tunnel: [w634 w638] -> w625
              frame False {
                # "No changes means we don't need to update anything"
              }
              frame True {
                # "Format the new shortcut\nto display in the combo box"
                n166 = for {
                  tunnel: w641 -> [w646] mode=indexing
                  tunnel: [w643] -> w640 mode=indexing
                  n167 = Index Array(array=w646) -> (element #1=w645:string, element #2=w644:string)  [unwired: 2 in]
                  n168 = Format Into String(format string="%s (%s)", w645, w644) -> (resulting string=w643:string)  [unwired: 2 in, 1 out]
                }
                n169 = Build Array (concatenate)(w640, w642) -> (w638:string[])
                n170 = local write "Shortcuts"(w640) -> ()
                n171 = property on="Object Name" class="CmbBox"("Value"="", "Key Focus"=TRUE) -> ()  [unwired: 2 in, 2 out]
                n172 = property on="Name Match List" class="LstBox (strict)"("Item Names"=w638, "Disabled Items"=i32[] []) -> ()  [unwired: 2 in, 2 out]
              }
            }
          }
          event "Object Name": Key Down?; "Object Name": event type 3.0.x8000000b {
            # "Whenever we have code that updates the Name Match List via local variable, we now need to also Val(Sgnl) the listbox so the code that updates the context help window can run."
            # "If Tab/Shift Tab is pressed, fake like Down/Up was pressed.  Otherwise, use the actual VKey value."
            # "Pressing Up, Down, Page Up, or Page Down in the Combo Box needs to be discarded so the Combo Box drop down doesn't show up.  However, we need to start navigating the listbox.  So the listbox selection is changed.  If the selection goes off-screen, we need to scroll it manually (that's what the TopRow call does)."
            n173 = event-data() -> ("VKey"=w652:T6, "Char"=w657:i16, "PlatMods.Shift"=w650:bool)  [unwired: 1 out]
            n174 = Equal?(x=eventvkey."ASCII", y=w652) -> (x = y?=w654:bool)
            n175 = Equal?(x=w657, y=i16 9 ("x")) -> (x = y?=w655:bool)
            n176 = And(x=w654, y=w655) -> (x .and. y?=w653:bool)
            n177 = case shown="True" w653 {
              tunnel: w652 -> [w664 _]
              tunnel: [w664 w665] -> w651
              tunnel: w650 -> [_ w668]
              frame False {
              }
              frame True {
                n178 = Select(t=eventvkey."Up" ("x"), s=w668, f=eventvkey."Down" ("x")) -> (s? t:f=w665:T6)
              }
            }
            n179 = case shown="\"PageDown\"" w651 {
              tunnel: w659 -> [_ w678 w707 w736 w761 _]
              tunnel: [FALSE TRUE TRUE TRUE TRUE w785] -> w661
              tunnel: w660 -> [_ w683 w712 w741 w766 _]
              tunnel: [TRUE FALSE FALSE FALSE FALSE w785] -> w648
              frame "ASCII", "Two Byte Char", Default {
                # "ASCII or multibyte key means the listbox needs to be updated"
                # "Up or Down was not pressed...assume the list was changed by a character or backspace keypress\nand rescroll the list to the top"
                n180 = property on="Name Match List" class="LstBox (strict)"("Top Row"=0) -> ()  [unwired: 2 in, 2 out]
              }
              frame "PageDown" {
                n181 = local read "Name Match List"() -> (w688:i32)
                n182 = Array Size(array=w683) -> (size(s)=w682:i32)
                n183 = property on="Name Match List" class="LstBox (strict)"() -> ("Top Row"=w679:i32)  [unwired: 2 in, 2 out]
                n184 = Decrement(x=w682) -> (x-1=w674:i32)
                n185 = To Long Integer(number=w678) -> (32bit integer=w673:i32)
                n186 = Add(x=w688, y=w673) -> (x+y=w676:i32)
                n187 = Greater?(x=w676, y=w674) -> (0:w677:bool)
                n188 = case shown="True" w677 {
                  tunnel: w676 -> [w689 _]
                  tunnel: [w689 w693] -> w675
                  tunnel: w674 -> [_ w691]
                  tunnel: w673 -> [_ w694]
                  frame False {
                  }
                  frame True {
                    n189 = Less?(x=w691, y=w694) -> (x < y?=w692:bool)
                    n190 = Select(t=w691, s=w692, f=0 ("y")) -> (s? t:f=w693:i32)
                  }
                }
                n191 = Add(x=w679, y=w673) -> (x+y=w687:i32)
                n192 = Decrement(x=w687) -> (x-1=w685:i32)
                n193 = In Range and Coerce(upper limit=w674, x=w675, lower limit=0 ("y")) -> (coerced(x)=w672:i32)  [unwired: 1 out]
                n194 = local write "Name Match List"(w672) -> ()
                n195 = In Range and Coerce(upper limit=w685, x=w672, lower limit=w679) -> (In Range?=w686:bool)  [unwired: 1 out]
                n196 = case shown="False" w686 {
                  tunnel: w672 -> [w695 _]
                  tunnel: w673 -> [w696 _]
                  frame False {
                    n197 = case shown="0" w695 {
                      selector: w695 -> [w698 w699]
                      tunnel: [w698 w702] -> w697
                      tunnel: w696 -> [_ w701]
                      frame 0 {
                      }
                      frame Default {
                        n198 = Subtract(x=w699, y=w701) -> (x-y=w700:i32)
                        n199 = Increment(x=w700) -> (x+1=w702:i32)
                      }
                    }
                    n200 = property on="Name Match List" class="LstBox (strict)"("Top Row"=w697) -> ()  [unwired: 2 in, 2 out]
                  }
                  frame True {
                    # "The newly selected item is visible, so no scrolling is necessary"
                  }
                }
              }
              frame "PageUp" {
                n201 = local read "Name Match List"() -> (w718:i32)
                n202 = Array Size(array=w712) -> (size(s)=w711:i32)
                n203 = property on="Name Match List" class="LstBox (strict)"() -> ("Top Row"=w708:i32)  [unwired: 2 in, 2 out]
                n204 = Decrement(x=w711) -> (x-1=w706:i32)
                n205 = To Long Integer(number=w707) -> (32bit integer=w704:i32)
                n206 = Subtract(x=w718, y=w704) -> (x-y=w705:i32)
                n207 = case shown="..-1" w705 {
                  selector: w705 -> [_ w724]
                  tunnel: [w720 w724] -> w714
                  tunnel: w706 -> [w721 _]
                  tunnel: w704 -> [w723 _]
                  frame ..-1 {
                    n208 = Less?(x=w721, y=w723) -> (x < y?=w722:bool)
                    n209 = Select(t=0, s=w722, f=w721) -> (s? t:f=w720:i32)
                  }
                  frame 0.. {
                  }
                }
                n210 = Add(x=w708, y=w704) -> (x+y=w717:i32)
                n211 = Decrement(x=w717) -> (x-1=w715:i32)
                n212 = In Range and Coerce(upper limit=w706, x=w714, lower limit=0 ("y")) -> (coerced(x)=w703:i32)  [unwired: 1 out]
                n213 = local write "Name Match List"(w703) -> ()
                n214 = In Range and Coerce(upper limit=w715, x=w703, lower limit=w708) -> (In Range?=w716:bool)  [unwired: 1 out]
                n215 = case shown="False" w716 {
                  tunnel: w708 -> [_ _]
                  tunnel: w703 -> [w727 _]
                  tunnel: w706 -> [w731 _]
                  tunnel: w704 -> [w730 _]
                  frame False {
                    n216 = Subtract(x=w731, y=w730) -> (x-y=w728:i32)
                    n217 = Greater?(x=w727, y=w728) -> (0:w729:bool)
                    n218 = Increment(x=w728) -> (x+1=w725:i32)
                    n219 = Select(t=w725, s=w729, f=w727) -> (s? t:f=w726:i32)
                    n220 = property on="Name Match List" class="LstBox (strict)"("Top Row"=w726) -> ()  [unwired: 2 in, 2 out]
                  }
                  frame True {
                    # "The newly selected item is visible, so no scrolling is necessary"
                  }
                }
              }
              frame "Down" {
                n221 = local read "Name Match List"() -> (w747:i32)
                n222 = Array Size(array=w741) -> (size(s)=w740:i32)
                n223 = property on="Name Match List" class="LstBox (strict)"() -> ("Top Row"=w737:i32)  [unwired: 2 in, 2 out]
                n224 = Decrement(x=w740) -> (x-1=w734:i32)
                n225 = To Long Integer(number=w736) -> (32bit integer=w735:i32)
                n226 = Equal?(x=w734, y=w747) -> (x = y?=w733:bool)
                n227 = case shown="True" w733 {
                  tunnel: [w749 0] -> w743
                  tunnel: w747 -> [w748 _]
                  frame False {
                    n228 = Increment(x=w748) -> (x+1=w749:i32)
                  }
                  frame True {
                  }
                }
                n229 = Add(x=w737, y=w735) -> (x+y=w746:i32)
                n230 = Decrement(x=w746) -> (x-1=w744:i32)
                n231 = In Range and Coerce(upper limit=w734, x=w743, lower limit=0 ("y")) -> (coerced(x)=w732:i32)  [unwired: 1 out]
                n232 = local write "Name Match List"(w732) -> ()
                n233 = In Range and Coerce(upper limit=w744, x=w732, lower limit=w737) -> (In Range?=w745:bool)  [unwired: 1 out]
                n234 = case shown="False" w745 {
                  tunnel: w737 -> [w753 _]
                  tunnel: w732 -> [w751 _]
                  frame False {
                    n235 = case shown="0" w751 {
                      tunnel: w753 -> [_ w756]
                      tunnel: [0 w755] -> w752
                      frame 0 {
                      }
                      frame Default {
                        n236 = Increment(x=w756) -> (x+1=w755:i32)
                      }
                    }
                    n237 = property on="Name Match List" class="LstBox (strict)"("Top Row"=w752) -> ()  [unwired: 2 in, 2 out]
                  }
                  frame True {
                    # "The newly selected item is visible, so no scrolling is necessary"
                  }
                }
              }
              frame "Up" {
                n238 = local read "Name Match List"() -> (w772:i32)
                n239 = Array Size(array=w766) -> (size(s)=w765:i32)
                n240 = property on="Name Match List" class="LstBox (strict)"() -> ("Top Row"=w762:i32)  [unwired: 2 in, 2 out]
                n241 = Decrement(x=w765) -> (x-1=w759:i32)
                n242 = To Long Integer(number=w761) -> (32bit integer=w760:i32)
                n243 = Decrement(x=w772) -> (x-1=w758:i32)
                n244 = case shown="..-1" w758 {
                  selector: w758 -> [_ w774]
                  tunnel: [w773 w774] -> w768
                  tunnel: w759 -> [w773 _]
                  frame ..-1 {
                  }
                  frame 0.. {
                  }
                }
                n245 = Add(x=w762, y=w760) -> (x+y=w771:i32)
                n246 = Decrement(x=w771) -> (x-1=w769:i32)
                n247 = In Range and Coerce(upper limit=w759, x=w768, lower limit=0 ("y")) -> (coerced(x)=w757:i32)  [unwired: 1 out]
                n248 = local write "Name Match List"(w757) -> ()
                n249 = In Range and Coerce(upper limit=w769, x=w757, lower limit=w762) -> (In Range?=w770:bool)  [unwired: 1 out]
                n250 = case shown="False" w770 {
                  tunnel: w762 -> [w778 _]
                  tunnel: w760 -> [w776 _]
                  tunnel: w759 -> [w775 _]
                  frame False {
                    n251 = case shown="..0" w778 {
                      selector: w778 -> [_ w783]
                      tunnel: [w779 w784] -> w777
                      tunnel: w776 -> [w781 _]
                      tunnel: w775 -> [w782 _]
                      frame ..0 {
                        n252 = Subtract(x=w782, y=w781) -> (x-y=w780:i32)
                        n253 = Increment(x=w780) -> (x+1=w779:i32)
                      }
                      frame 1.. {
                        n254 = Decrement(x=w783) -> (x-1=w784:i32)
                      }
                    }
                    n255 = property on="Name Match List" class="LstBox (strict)"("Top Row"=w777) -> ()  [unwired: 2 in, 2 out]
                  }
                  frame True {
                    # "The newly selected item is visible, so no scrolling is necessary"
                  }
                }
              }
              frame "Shift".."Cmd" {
                w785 = FALSE
                # "Shift should not trigger the bottom loop to do a search."
              }
            }
            n256 = flat-sequence "For updating context help" {
              tunnel: w648 -> [_]
              frame #0 {
                n257 = local read "Name Match List"() -> (w663:i32)
                n258 = property on="Name Match List" class="LstBox (strict)"("Val(Sgnl)"=w663) -> ()  [unwired: 2 in, 2 out]
              }
            }
            n259 = event-data("Discard?"=w661) -> ()  [unwired: 1 in, 1 out]
          }
          event Timeout {
            # "The Context Help window is easily excitable, in that if you hover over controls, it tries to display their context help. Well, we don't want it to display the context help of Quick Drop controls, we want it to display the context help of the currently-selected item in Quick Drop. By updating the context help 100 times per second, it never gets a chance to update with the QD UI context help. Since there appears to be a built-in delay in context help, we never see any flicker either."
            n260 = event-data() -> ()  [unwired: 2 out]
            n261 = local read "context help name"() -> (w786:string)
            n262 = case shown="True" w790 {
              tunnel: w791 -> [_ w801]
              frame False {
                # "No need to update the listbox"
              }
              frame True {
                # "Remove empties and pass to bottom loop"
                # "convert to array\n(space-delimited)"
                n263 = property on="Object Name" class="CmbBox"() -> ("Text.Text"=w794:string)  [unwired: 2 in, 2 out]
                n264 = case shown="Default" w794 {
                  frame Default {
                  }
                  frame "" {
                    n265 = property on="Name Match List" class="LstBox (strict)"("Value"=-1 ("Name Match List")) -> ()  [unwired: 2 in, 2 out]
                  }
                }
                n266 = To Lower Case(string=w794) -> (all lower case string=w798:string)
                n267 = Spreadsheet String To Array(delimiter (Tab)=" ", format string="%s", spreadsheet string=w798, array type (2D Dbl)=string[] []) -> (array=w796:string[])
                n268 = for {
                  tunnel: w796 -> [w805] mode=indexing
                  tunnel: [w805] -> w795 mode=indexing if=w803
                  n269 = Empty String/Path?(string/path=w805) -> (empty?=w804:bool)
                  n270 = Not(x=w804) -> (.not. x?=w803:bool)
                }
                n271 = Enqueue Element(queue=w801, element=w795) -> ()  [unwired: 1 in, 4 out]
              }
            }
            n272 = invoke class="App" method="UI.ShowPaletteObjContextHelp"("Name"=w786) -> ()  [unwired: 3 in, 4 out]
          }
          event User Event {
            # "Whenever we have code that updates the Name Match List, we now need to Val(Sgnl) the listbox so the code that updates the context help window can run."
            # "The name matching is done... update the listbox with the new matched names"
            n273 = event-data() -> ("Matched Names"=w820:string[])  [unwired: 1 out]
            n274 = local read "Name Match List"() -> (w813:i32)
            n275 = property on="Name Match List" class="LstBox (strict)"() -> ("Item Names"=w825:string[])  [unwired: 2 in, 2 out]
            n276 = Greater Or Equal To 0?(x=w813) -> (x >= 0?=w814:bool)
            n277 = Select(t=w813, s=w814, f=0) -> (s? t:f=w811:i32)
            n278 = property on="Object Name" class="CmbBox"() -> ("Text.Text"=w807:string)  [unwired: 2 in, 2 out]
            n279 = Empty Array?(array=w820) -> (empty?=w827:bool)
            n280 = To Lower Case(string=w807) -> (all lower case string=w823:string)
            n281 = To Lower Case(string=w820) -> (all lower case string=w822:string[])
            n282 = Search 1D Array(1D array=w822, element=w823) -> (index of element=w824:i32)  [unwired: 1 in]
            n283 = case shown="-1" w824 {
              selector: w824 -> [w829 _]
              tunnel: [w829 w830] -> w819
              tunnel: w823 -> [_ w831]
              tunnel: w822 -> [_ w834]
              frame Default {
                # "What's currently typed exactly matches something in the list, regardless of position. Use that."
              }
              frame -1 {
                w830 = 0 ("f")
                # "Always pick the top item of the list. New in 2020."
                n284 = for {
                  tunnel: w834 -> [w838] mode=indexing
                  tunnel: [w842] -> w833
                  tunnel: [w835] -> w832
                  tunnel: w831 -> [w839]
                  i -> [w842]
                  stop <- w836 stop-if-true
                  n285 = Match Pattern(string=w838, regular expression=" (") -> (offset past match=w840:i32)  [unwired: 1 in, 3 out]
                  n286 = case shown="Default" w840 {
                    tunnel: [FALSE TRUE] -> w837
                    tunnel: w839 -> [w847 _]
                    tunnel: w838 -> [w849 _]
                    tunnel: [w843 FALSE] -> w835
                    frame Default {
                      n287 = Format Into String(format string="^%s (", w847) -> (resulting string=w845:string)  [unwired: 2 in, 1 out]
                      n288 = Match Pattern(string=w849, regular expression=w845) -> (offset past match=w844:i32)  [unwired: 1 in, 3 out]
                      n289 = Greater Or Equal To 0?(x=w844) -> (x >= 0?=w843:bool)
                    }
                    frame -1 {
                      # "no more shortcuts, and we never found a shortcut match"
                    }
                  }
                  n290 = Or(x=w835, y=w837) -> (x .or. y?=w836:bool)
                }
                n291 = Select(t=w833, s=w832, f=w830) -> ()  [unwired: 1 out]
              }
            }
            n292 = case shown="False" w827 {
              tunnel: w826 -> [_ w863]
              tunnel: w825 -> [_ w862]
              tunnel: [w855 w860] -> w816
              tunnel: w820 -> [w852 _]
              tunnel: [w853 -1 ("f")] -> w810
              tunnel: w819 -> [w853 _]
              tunnel: [_ i32[] [0] ("Disabled Items")] -> w818
              tunnel: [w852 w857] -> w817
              tunnel: w811 -> [w854 w856]
              frame False {
                # "Save the first match in case there are no matches later"
                n293 = Index Array(array=w852, index=w854) -> (element=w855:string)
                n294 = property on="Name Match List" class="LstBox (strict)"("Top Row"=w853) -> ()  [unwired: 2 in, 2 out]
              }
              frame True {
                # "Nothing matched...pull the first item prior to no matches, and put it in the list disabled"
                n295 = Empty Array?(array=w862) -> (empty?=w864:bool)
                n296 = Index Array(array=w862, index=w856) -> (element=w861:string)
                n297 = Select(t=w863, s=w864, f=w861) -> (s? t:f=w860:string)
                n298 = Build Array(w860) -> (w857:string[])
              }
            }
            n299 = Empty String/Path?(string/path=w807) -> (empty?=w808:bool)
            n300 = Select(t=-1, s=w808, f=w810) -> (s? t:f=w806:i32)
            n301 = property on="Name Match List" class="LstBox (strict)"("Item Names"=w817, "Disabled Items"=w818) -> ()  [unwired: 2 in, 2 out]
            n302 = property on="Name Match List" class="LstBox (strict)"("Val(Sgnl)"=w806) -> ()  [unwired: 2 in, 2 out]
          }
          event Panel Resize {
            # "When the panel is resized, the combo box will automatically resize,\nbut we need to programmatically resize the decoration surrounding it."
            n303 = event-data() -> ()  [unwired: 2 out]
            n304 = property on="Object Name" class="CmbBox"() -> (error out=w869:errorcluster, "Width"=w871:u32)  [unwired: 2 in, 1 out]
            n305 = Subtract(x=w871, y=u32 5) -> (x-y=w872:u32)
            n306 = property class="Decor"(reference=w870, error in=w869, "Width"=w872, "Left"=1) -> (error out=w866:errorcluster)  [unwired: 1 out]
            n307 = property on="Name Match List" class="LstBox (strict)"(error in=w866) -> ("Number of Rows"=w867:u32)  [unwired: 1 in, 2 out]
          }
          event "Name Match List": Value Change {
            # "Whenever the value of the listbox changes, we need to update the context help with help for the item currently selected. This code first tries to match the name exactly. If it does, great. If not, this must be a shortcut, so the name of the object needs to be extracted from the parenthetical at the end of the string."
            n308 = event-data() -> ("NewVal"=w884:i32)  [unwired: 1 out]
            n309 = case shown="Default" w884 {
              selector: w884 -> [w895 _]
              tunnel: w881 -> [w893 _]
              tunnel: w880 -> [w894 _]
              tunnel: [w890 _] -> w878
              frame Default {
                # "Valid value selected in listbox"
                n310 = Index Array(array=w894, index=w895) -> (element=w891:string)
                n311 = Search 1D Array(1D array=w893, element=w891) -> (index of element=w892:i32)  [unwired: 1 in]
                n312 = case shown="Default" w892 {
                  tunnel: [w896 w902] -> w890
                  tunnel: w891 -> [w896 w903]
                  frame Default {
                    # "Listbox entry exactly matches a palette item name. Use it."
                  }
                  frame -1 {
                    # "extract item name from parenthesis after shortcut"
                    n313 = Match Pattern(string=w903, regular expression="(.*)$") -> (match substring=w897:string)  [unwired: 1 in, 3 out]
                    n314 = String Length(string=w897) -> (length=w900:i32)
                    n315 = Subtract(x=w900, y=2) -> (x-y=w898:i32)
                    n316 = String Subset(string=w897, offset (0)=1, length (rest)=w898) -> (substring=w902:string)
                  }
                }
              }
              frame -1 {
                # "No valid value selected in the listbox"
              }
            }
            n317 = case shown="Default" w878 {
              selector: w878 -> [_ w887]
              tunnel: [_ w886] -> w877
              frame "" {
              }
              frame Default {
                # "Strip library from end"
                n318 = Match Pattern(string=w887, regular expression="\\[.*\\]$") -> (before substring=w889:string)  [unwired: 1 in, 3 out]
                n319 = call <vilib>:"Trim Whitespace.vi"("string"=w889) -> ("trimmed string"=w886:string)  [unwired: 1 in]
              }
            }
            "context help name" <- w877
          }
        }
      }
      n320 = while {
        tunnel: w303 -> [w318]
        tunnel: w302 -> [w316]
        tunnel: w299 -> [w315]
        tunnel: w297 -> [w314]
        tunnel: w287 -> [w312]
        tunnel: w281 -> [w311]
        tunnel: w280 -> [w310]
        tunnel: w286 -> [w309]
        tunnel: w282 -> [w308]
        tunnel: w271 -> [w307]
        stop <- w313 stop-if-true
        n321 = Dequeue Element(queue=w318) -> (element=w317:string[], error out=w313:errorcluster)  [unwired: 1 in, 3 out]
        n322 = case shown="No Error" w313 {
          tunnel: w317 -> [w329 _]
          tunnel: w316 -> [w328 _]
          tunnel: w315 -> [w327 _]
          tunnel: w314 -> [w320 _]
          tunnel: w312 -> [w325 _]
          tunnel: w311 -> [w324 _]
          tunnel: w310 -> [w323 _]
          tunnel: w309 -> [w322 _]
          tunnel: w308 -> [w321 _]
          tunnel: w307 -> [w319 _]
          frame No Error {
            # "Fire User Event once the matching is done so the listbox can be updated"
            n323 = Empty Array?(array=w329) -> (empty?=w330:bool)
            n324 = case shown="False" w330 {
              tunnel: w329 -> [w335 _]
              tunnel: [w332 w381] -> w326
              tunnel: w328 -> [w351 _]
              tunnel: w327 -> [w346 _]
              tunnel: w325 -> [w356 _]
              tunnel: w324 -> [w354 _]
              tunnel: w323 -> [w355 _]
              tunnel: w322 -> [w353 _]
              tunnel: w321 -> [w347 _]
              tunnel: w319 -> [w336 w381]
              frame False {
                # ">>Class Matches>>"
                # "Take what is typed and see if it matches any of the search results exactly from the beginning of the string. If so, put those results at the very top of the list, regardless of result type."
                # ">>ProjectItem Matches>>"
                # ">>Shorcuts Matches>>"
                n325 = case shown="No Error" w356 {
                  tunnel: w355 -> [w365 _]
                  tunnel: w354 -> [w366 _]
                  tunnel: w335 -> [w367 _]
                  tunnel: w353 -> [w364 _]
                  tunnel: [w363 _] -> w350
                  tunnel: w347 -> [w362 _]
                  tunnel: w346 -> [w361 _]
                  frame No Error {
                    n326 = case shown="True" w362 {
                      tunnel: w367 -> [w377 w379]
                      tunnel: w366 -> [w371 _]
                      tunnel: w365 -> [w372 _]
                      tunnel: w364 -> [w370 _]
                      tunnel: [w373 w380] -> w363
                      tunnel: w361 -> [_ w378]
                      frame False {
                        n327 = Array To Spreadsheet String(delimiter (Tab)=" " ("format string"), array=w377, 3:"%s" ("format string")) -> (spreadsheet string=w375:string)
                        n328 = call <vilib>:"Trim Whitespace.vi"("string"=w375) -> ("trimmed string"=w369:string)  [unwired: 1 in]
                        n329 = invoke class="App" method="SearchSyncSearchForQD"(reference=w372, "SessionID"=w371, "MaxResults"=u32 100, "Query"=w369, "isOnFrontPanel"=w370) -> ("Results"=w373:string[])  [unwired: 3 in, 7 out]
                      }
                      frame True {
                        n330 = call "OldSearchAlgorithm.vi"("Query terms"=w379, "SearchList Case"=w378) -> ("Search Result"=w380:string[])  [unwired: 9 in]
                      }
                    }
                  }
                  frame Error {
                  }
                }
                n331 = property on="Object Name" class="CmbBox"() -> ("Text.Text"=w337:string)  [unwired: 2 in, 2 out]
                n332 = local read "Shortcuts"() -> (w352:string[])
                n333 = case shown="Default" w337 {
                  tunnel: w336 -> [w357 w359]
                  tunnel: [w357 w360] -> w331
                  tunnel: w335 -> [_ w358]
                  frame "" {
                  }
                  frame Default {
                    n334 = call "OldSearchAlgorithm.vi"("Query terms"=w358, "SearchList Case"=w359) -> ("Search Result"=w360:string[])  [unwired: 9 in]
                  }
                }
                n335 = call "OldSearchAlgorithm.vi"("Query terms"=w335, "SearchList Case"=w352) -> ("Search Result"=w349:string[])  [unwired: 9 in]
                n336 = call "OldSearchAlgorithm.vi"("Query terms"=w335, "SearchList Case"=w351) -> ("Search Result"=w348:string[])  [unwired: 9 in]
                n337 = Build Array (concatenate)(w349, w350, w348) -> (w333:string[])
                n338 = Array To Spreadsheet String(delimiter (Tab)=" ", array=w335, 3:"%s") -> (spreadsheet string=w341:string)
                n339 = Match Pattern(string=w341, regular expression="^[\\t\\n\\r\\s]*") -> (after substring=w339:string)  [unwired: 1 in, 3 out]
                n340 = Match Pattern(string=w339, regular expression="[\\t\\n\\r\\s]*$") -> (before substring=w338:string)  [unwired: 1 in, 3 out]
                n341 = Concatenate Strings("^", w338) -> (w334:string)
                n342 = call "Sort Matches.vi"("Filter"=w334, "Matches"=w333, "Class Matches"=w331) -> ("Filterd Matches"=w332:string[])
              }
              frame True {
              }
            }
            n343 = Generate User Event(user event=w320, event data cluster=w326) -> ()  [unwired: 2 in, 2 out]
          }
          frame Error {
          }
        }
      }
      n344 = Release Queue(queue=w300, force destroy? (F)=w301) -> ()  [unwired: 1 in, 3 out]
    }
    frame #4 {
      n345 = Empty Array?(array=w909) -> (empty?=w907:bool)
      n346 = case shown="False" w907 {
        tunnel: w911 -> [w926 _]
        tunnel: [w925 w939] -> w910
        tunnel: w909 -> [w924 _]
        tunnel: w906 -> [_ w939]
        tunnel: w905 -> [w923 _]
        frame False {
          n347 = case shown="False" w923 {
            tunnel: w926 -> [w930 w938]
            tunnel: [w929 w938] -> w925
            tunnel: w924 -> [w927 _]
            frame False {
              # "See if what's currently typed exactly matches something in the list, regardless of position. If so, use that. Otherwise, use the top item in the list."
              n348 = To Lower Case(string=w927) -> (all lower case string=w932:string[])
              n349 = To Lower Case(string="Object Name") -> (all lower case string=w933:string)
              n350 = Search 1D Array(1D array=w932, element=w933) -> (index of element=w931:i32)  [unwired: 1 in]
              n351 = case shown="Default" w931 {
                selector: w931 -> [w936 _]
                tunnel: w930 -> [_ w937]
                tunnel: [w934 w937] -> w929
                tunnel: "Object Name" -> [_ _]
                tunnel: w927 -> [w935 _]
                frame Default {
                  n352 = Index Array(array=w935, index=w936) -> (element=w934:string)
                }
                frame -1 {
                }
              }
            }
            frame True {
              # "The TRUE value coming in to this case indicates that this was a \"deliberate\" choice in the Quick Drop UI, so we shouldn't do any of the special code in the FALSE case that tries to make a better selection than what was specified. This case runs if:\n\n1. The user double-clicked in the list.\n2. The user pressed Enter, and the listbox had a non-initial value selected.\n3. The user Super Quick Dropped, and the listbox had a non-initial value selected."
            }
          }
        }
        frame True {
          # "If there are no results, use the last top result that we did have"
        }
      }
      n353 = Close Reference(reference=w913) -> ()  [unwired: 1 in, 1 out]
      n354 = property class="VI"() -> (error out=w918:errorcluster, "Front Panel.WinBounds"=w919:T5)  [unwired: 2 in, 1 out]
      n355 = case shown="False" w912 {
        tunnel: w915 -> [w941 _]
        tunnel: w914 -> [w940 _]
        frame False {
          n356 = invoke class="App" method="SearchCloseSession"(reference=w941, "SessionID"=w940) -> ()  [unwired: 2 in, 4 out]
        }
        frame True {
        }
      }
      n357 = invoke class="VI" method="FP.Close"(error in=w918) -> ()  [unwired: 2 in, 3 out]
    }
    frame #5 {
      w942 = "QuickDropPosition" ("Name")
      n358 = Equal?(x=w943, y=w951) -> (x = y?=w950:bool)
      n359 = case shown="False" w950 {
        tunnel: w943 -> [w970 _]
        tunnel: [w963 _] -> w947
        tunnel: w942 -> [w962 _]
        frame False {
          # "Bounds changed...write new bounds\nto Global Data and to INI file"
          n360 = Unbundle(w970) -> ("Left"=w969:i16, "Top"=w968:i16, "Right"=w967:i16, "Bottom"=w966:i16)
          n361 = Format Into String(format string="%d,%d,%d,%d", w969, w968, w967, w966) -> (resulting string=w964:string)  [unwired: 2 in, 1 out]
          n362 = call-by-ref "?"("value"=w964, "key"=w962) -> (error out=w963:errorcluster)  [unwired: 3 in, 6 out]
        }
        frame True {
          # "Bounds didn't change while window was\nopen...don't do anything"
        }
      }
      n363 = invoke class="App" method="Global Data.Set"("index"=w942, "value"=w943) -> ()  [unwired: 3 in, 5 out]
      n364 = case shown="False" w948 {
        tunnel: w953 -> [w956 _]
        tunnel: w952 -> [w961 _]
        tunnel: w944 -> [w960 _]
        tunnel: w945 -> [w958 _]
        tunnel: w949 -> [w959 _]
        tunnel: w947 -> [_ _]
        tunnel: w946 -> [w957 _]
        frame False {
          n365 = local read "Shortcuts"() -> (w955:string[])
          n366 = call "QuickDrop Process Drop Information.vi"("Listbox Contents"=w957, "Project Item Refs"=w958, "Project Items"=w959, "App Refnum"=w960, "Shortcut Info"=w961, "Text.Text"=w956, "Shortcuts"=w955, "Run for Plugin?"=FALSE ("Run from Plugin?")) -> ()  [unwired: 6 in, 2 out]
        }
        frame True {
        }
      }
    }
  }
  n367 = Close Reference(reference=w11) -> ()  [unwired: 1 in, 1 out]
  n368 = Close Reference(reference=w12) -> ()  [unwired: 1 in, 1 out]
